vi "LSM9DS1_Read.vi"(0 "LSM9DS1DevRef":T1={"DevStatus"={"status"=FALSE, "code"=0, "source"=""}, "Gyro Offset"={"Xzero"=0.0, "Yzero"=0.0, "Zzero"=0.0}, "StdDev Rates"={"Xsdo"=0.0, "Ysdo"=0.0, "Zsdo"=0.0}, "Reset"=FALSE, "Accel Offset"={"Xzero"=0.0, "Yzero"=0.0, "Zzero"=0.0}, "Motion Thresh"=0.0, "Mag Offset"={"Xzero"=0.0, "Yzero"=0.0, "Zzero"=0.0}, "I2C Bus"=enum."I2C On-Board", "Handle"=0, "Anomaly Thresh"=0.0, "Local Mag"=0.0, "Accel/Gyro_Address"=enum."0x6B", "Accel_Range"=enum."±4g", "Gyro_Range"=enum."±500dps", "Mag_Range"=enum."±2 gauss", "Mag_Address"=enum."0x1E", "accel_active"=FALSE, "gyro_active"=FALSE, "mag_active"=FALSE}, 9 "Reset":bool, 11 "error in (no error)":errorcluster) -> (3 "Filt_Pitch":dbl, 4 "LSM9DS1DevRef Out":T1={"DevStatus"={"status"=FALSE, "code"=0, "source"=""}, "Gyro Offset"={"Xzero"=0.0, "Yzero"=0.0, "Zzero"=0.0}, "StdDev Rates"={"Xsdo"=0.0, "Ysdo"=0.0, "Zsdo"=0.0}, "Reset"=FALSE, "Accel Offset"={"Xzero"=0.0, "Yzero"=0.0, "Zzero"=0.0}, "Motion Thresh"=0.0, "Mag Offset"={"Xzero"=0.0, "Yzero"=0.0, "Zzero"=0.0}, "I2C Bus"=enum."I2C On-Board", "Handle"=0, "Anomaly Thresh"=0.0, "Local Mag"=0.0, "Accel/Gyro_Address"=enum."0x6B", "Accel_Range"=enum."±4g", "Gyro_Range"=enum."±500dps", "Mag_Range"=enum."±2 gauss", "Mag_Address"=enum."0x1E", "accel_active"=FALSE, "gyro_active"=FALSE, "mag_active"=FALSE}, 6 "Gyro":T6, 8 "Accel":T5, 10 "Mag":T4, 15 "error out":errorcluster)   [LabVIEW 2015]
uses:
  <vilib>/Rock Robotics/WPI/I2C/WPI_I2CDevRef.ctl
  <vilib>/Rock Robotics/SystemInterfaces/i2clib/i2c_bus.ctl
  Gyro_TypeDef.ctl
  Accel_TypeDef.ctl
  Mag_TypeDef.ctl
  LSM9DS1DevRef.ctl
panel:
  out "Pitch 2":cluster{"Pitch":dbl, dbl}(graph)
  in  "FIlt_Fact":dbl=1.0
  in  "Filt_Fact":dbl
  in  "In":dbl=0.1
  out "Roll":dbl(knob) scale=-180.0..180.0
  out "Pitch":dbl(knob) scale=-90.0..90.0
  in  "I2CDevRef":T3={"DevStatus"={"status"=FALSE, "code"=0, "source"=""}, "Device Address"=0, "Handle"=0, "I2C Bus"=enum."Invalid"} {"Device Address" format="%.0x"}
  in  "I2CDevRef":T3={"DevStatus"={"status"=FALSE, "code"=0, "source"=""}, "Device Address"=0, "Handle"=0, "I2C Bus"=enum."Invalid"} {"Device Address" format="%.0x"}
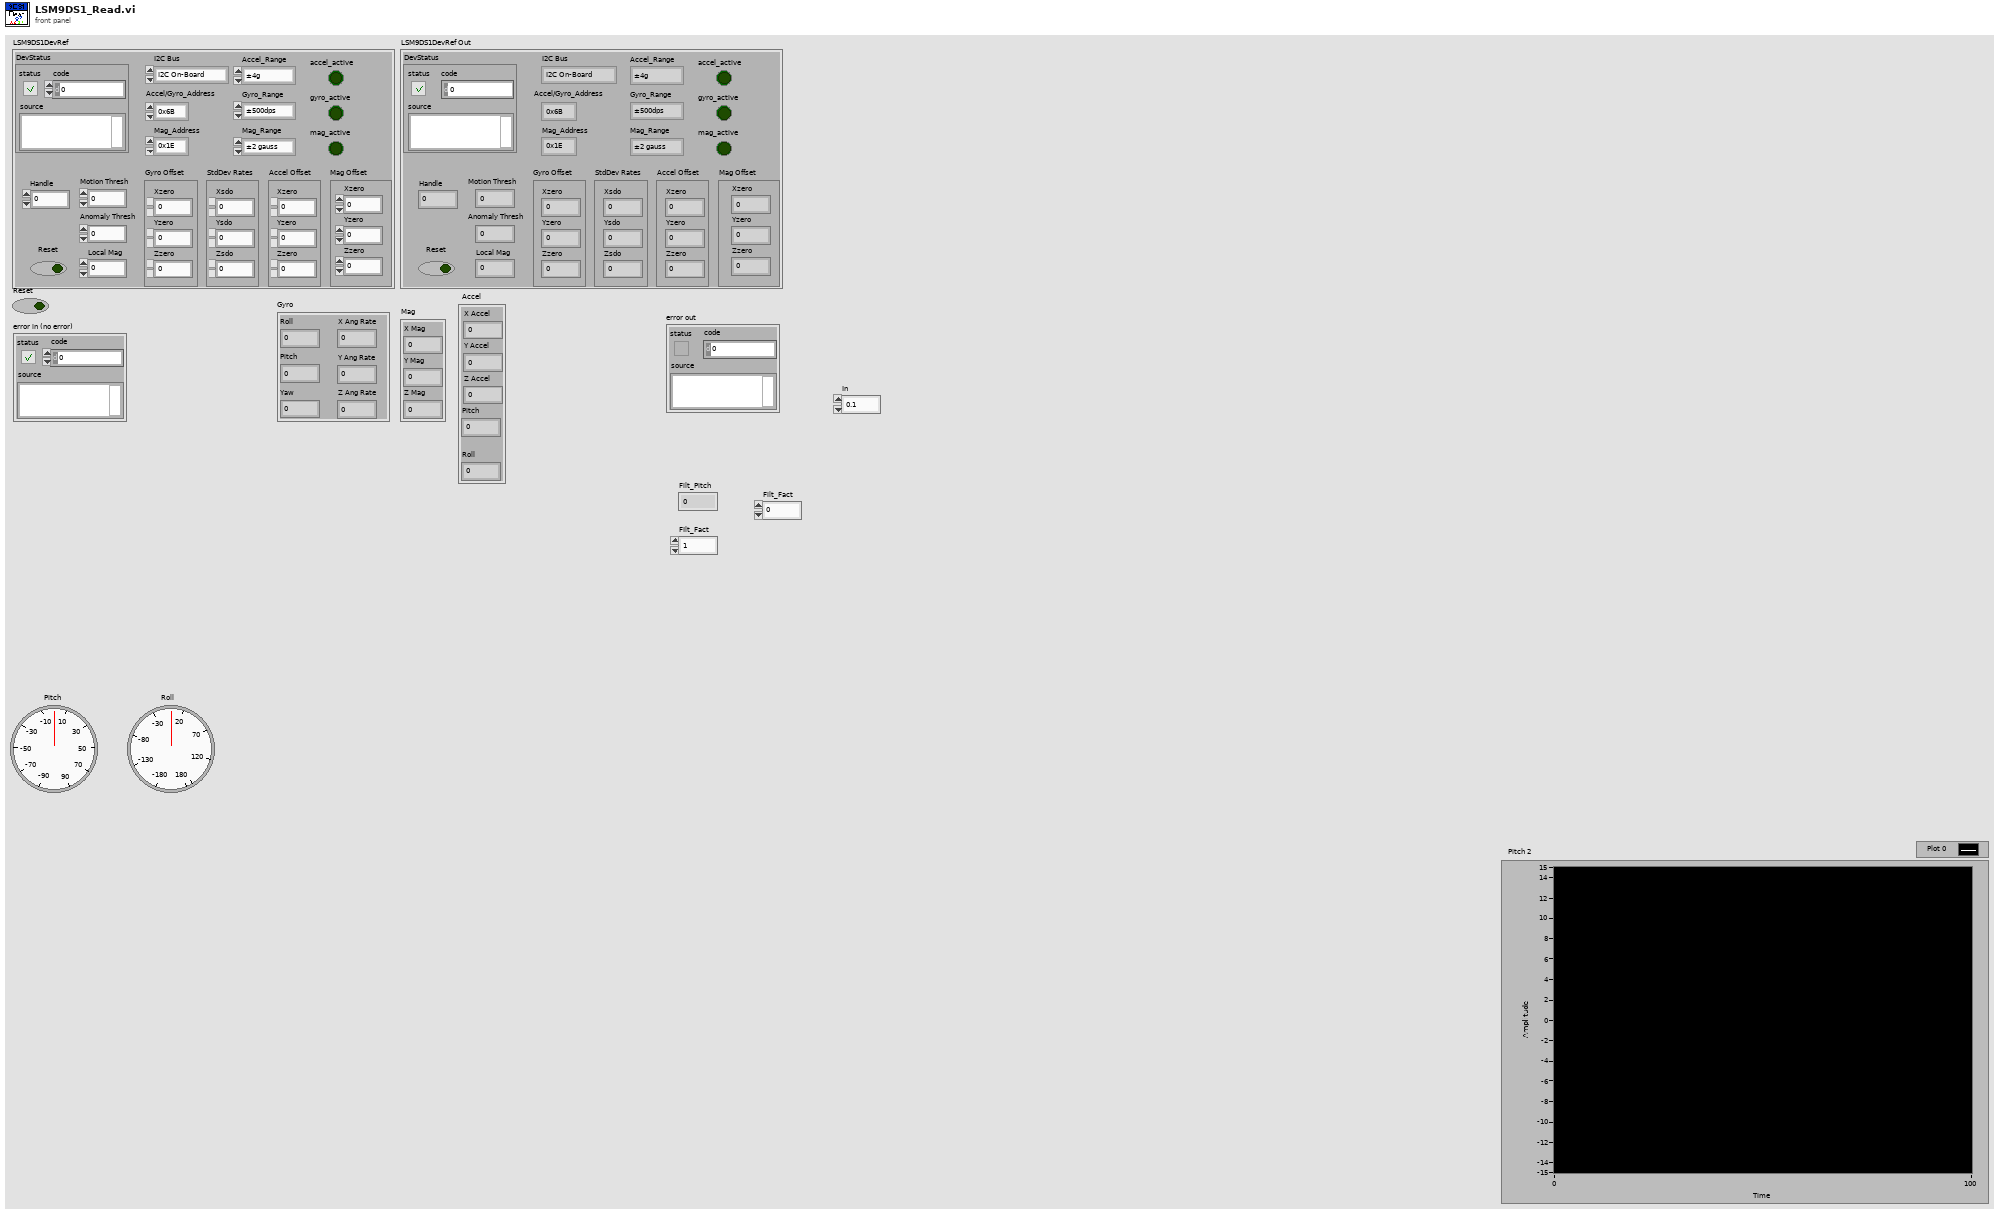
[diagram p1: front panel]
types:
  T1 = typedef "LSM9DS1DevRef.ctl" = cluster{"DevStatus":errorcluster, "Gyro Offset":cluster{"Xzero":dbl, "Yzero":dbl, "Zzero":dbl}, "StdDev Rates":cluster{"Xsdo":dbl, "Ysdo":dbl, "Zsdo":dbl}, "Reset":bool, "Accel Offset":cluster{"Xzero":dbl, "Yzero":dbl, "Zzero":dbl}, "Motion Thresh":dbl, "Mag Offset":cluster{"Xzero":dbl, "Yzero":dbl, "Zzero":dbl}, "I2C Bus":T2, "Handle":i32, "Anomaly Thresh":dbl, "Local Mag":dbl, "Accel/Gyro_Address":enum8{"0x6A", "0x6B"}, "Accel_Range":enum16{"±2g", "±16g", "±4g", "±8g", "disabled"}, "Gyro_Range":enum16{"±245dps", "±500dps", "disabled", "±2000dps"}, "Mag_Range":enum16{"±2 gauss", "±4 gauss", "±8 gauss", "±16 gauss", "disabled"}, "Mag_Address":enum8{"0x1C", "0x1E"}, "accel_active":bool, "gyro_active":bool, "mag_active":bool}
  T2 = typedef "i2c_bus.ctl" = enum16{"I2C On-Board", "I2C MXP", "Invalid"}
  T3 = typedef "WPI_I2CDevRef.ctl" = cluster{"DevStatus":errorcluster, "Device Address":u8, "Handle":i32, "I2C Bus":T2}
  T4 = typedef "Mag_TypeDef.ctl" = cluster{"X Mag":dbl, "Y Mag":dbl, "Z Mag":dbl}
  T5 = typedef "Accel_TypeDef.ctl" = cluster{"X Accel":dbl, "Y Accel":dbl, "Z Accel":dbl, "Pitch":dbl, "Roll":dbl}
  T6 = typedef "Gyro_TypeDef.ctl" = cluster{"Pitch":dbl, "Yaw":dbl, "X Ang Rate":dbl, "Y Ang Rate":dbl, "Z Ang Rate":dbl, "Roll":dbl}
  T7 = enum16{"±2 gauss", "±4 gauss", "±8 gauss", "±16 gauss", "disabled"}
  T8 = enum16{"±245dps", "±500dps", "disabled", "±2000dps"}
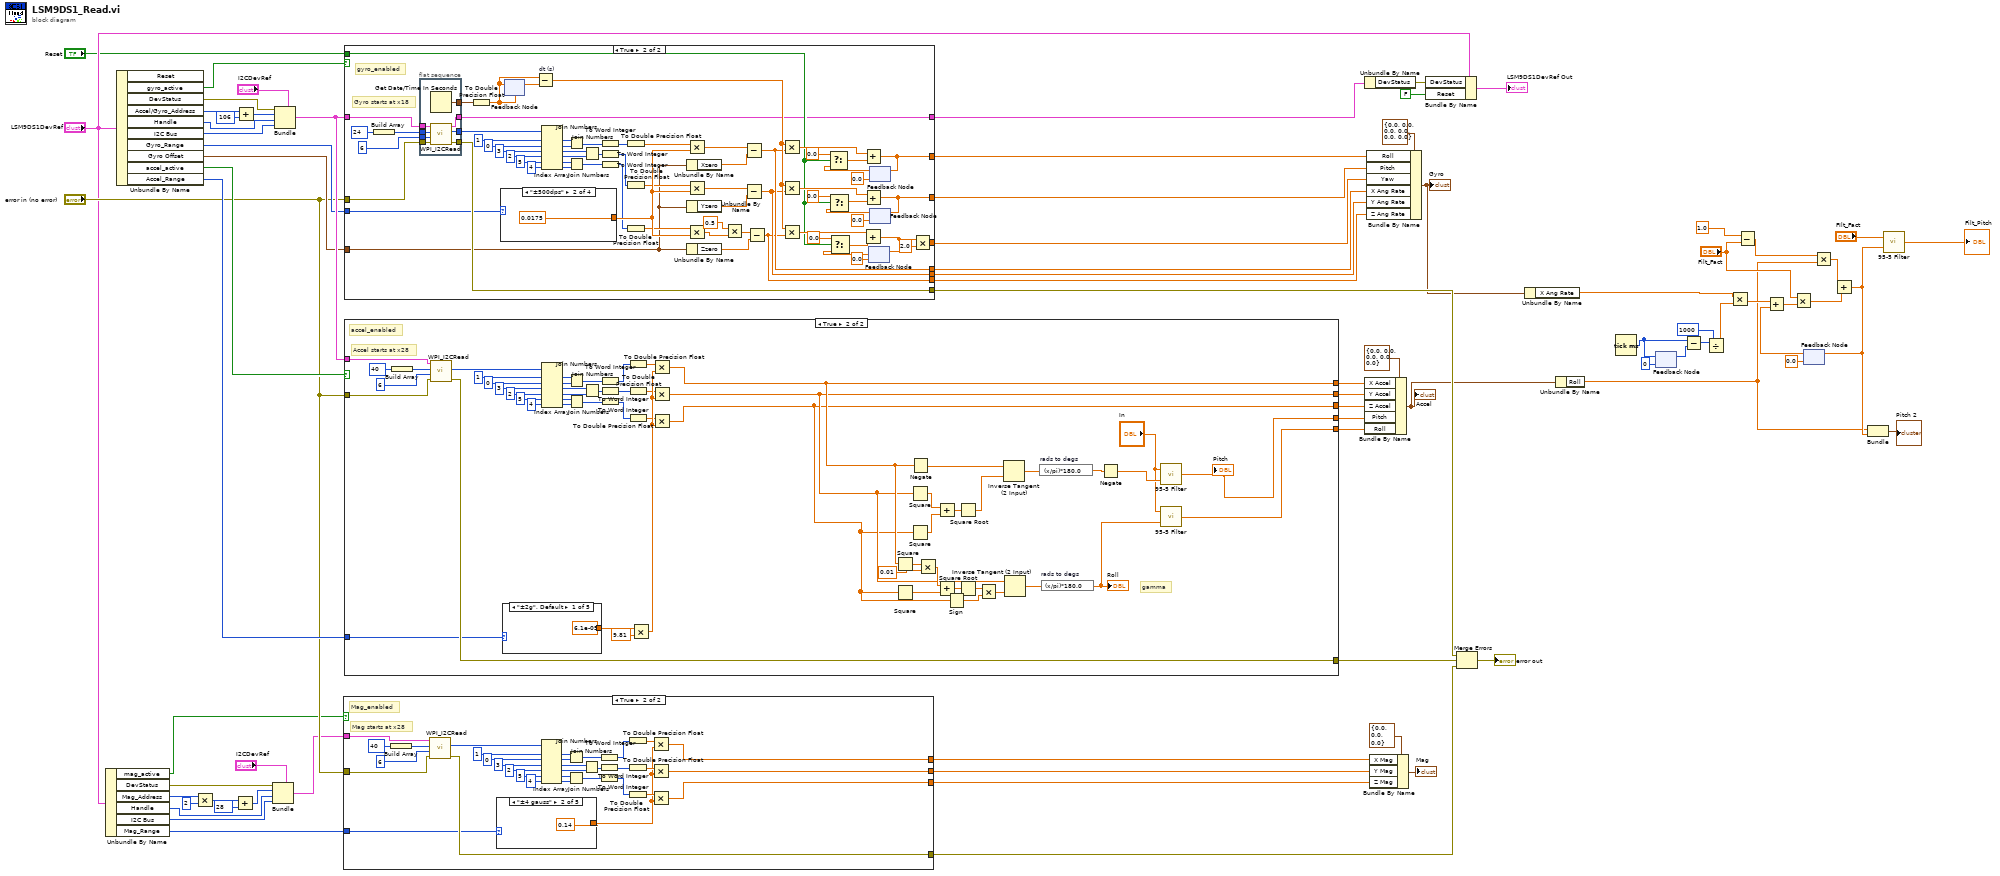
[diagram p0: block diagram]
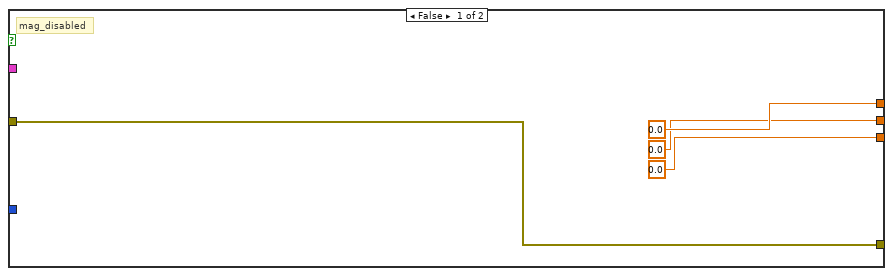
[diagram p2: hidden frame]
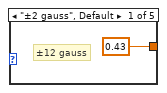
[diagram p3: hidden frame]
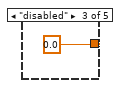
[diagram p4: hidden frame]
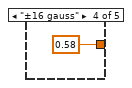
[diagram p5: hidden frame]
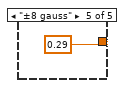
[diagram p6: hidden frame]
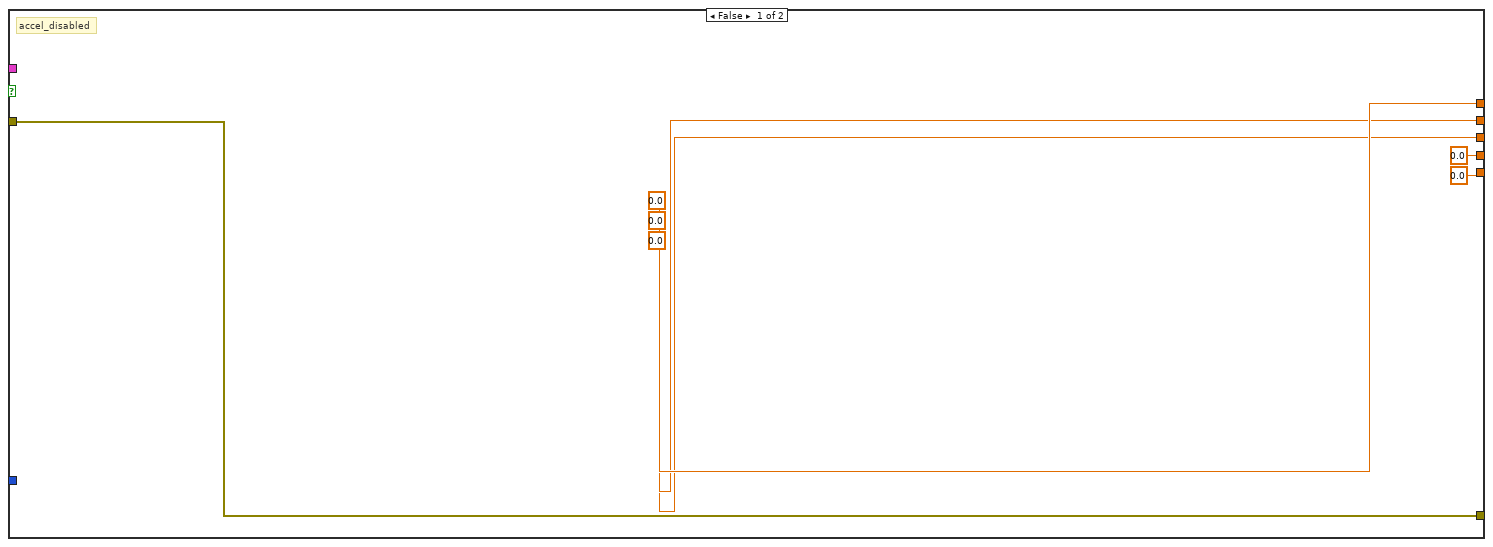
[diagram p7: hidden frame]
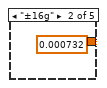
[diagram p8: hidden frame]
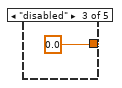
[diagram p9: hidden frame]
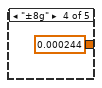
[diagram p10: hidden frame]
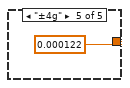
[diagram p11: hidden frame]
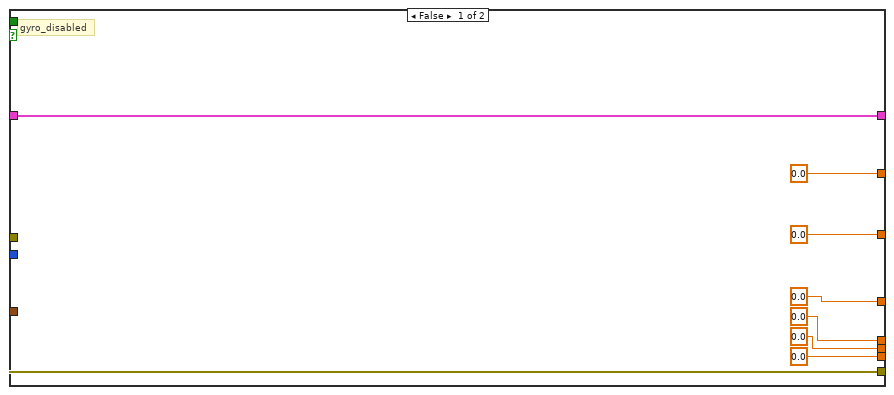
[diagram p12: hidden frame]
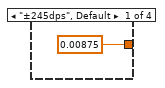
[diagram p13: hidden frame]
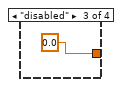
[diagram p14: hidden frame]
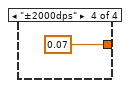
[diagram p15: hidden frame]
diagram:
  n1 = Unbundle By Name("LSM9DS1DevRef") -> ("mag_active"=w42:bool, "DevStatus"=w37:errorcluster, "Mag_Address"=w36:enum8{"0x1C", "0x1E"}, "Handle"=w35:i32, "I2C Bus"=w33:T2, "Mag_Range"=w44:T7)
  n2 = Unbundle By Name("LSM9DS1DevRef") -> ("gyro_active"=w49:bool, "DevStatus"=w56:errorcluster, "Accel/Gyro_Address"=w57:enum8{"0x6A", "0x6B"}, "Handle"=w54:i32, "I2C Bus"=w53:T2, "Gyro_Range"=w50:T8, "Gyro Offset"=w48:cluster{"Xzero":dbl, "Yzero":dbl, "Zzero":dbl}, "accel_active"=w47:bool, "Accel_Range"=w46:enum16{"±2g", "±16g", "±4g", "±8g", "disabled"})  [unwired: 1 out]
  n3 = Multiply(x=w36, y=u8 2) -> (x*y=w40:u8)
  n4 = Add ("Gyro/Accel Slave Address")(x=w40, y=u8 28) -> (x+y=w34:u8)
  n5 = Add ("Gyro/Accel Slave Address")(x=w57, y=u8 106) -> (x+y=w55:u8)
  n6 = Bundle(cluster="I2CDevRef", "DevStatus"=w37, "Device Address"=w34, "Handle"=w35, "I2C Bus"=w33) -> (w41:T3)
  n7 = Bundle(cluster="I2CDevRef", "DevStatus"=w56, "Device Address"=w55, "Handle"=w54, "I2C Bus"=w53) -> (w51:T3)
  n8 = case shown="True" w42 {
    tunnel: [0.0 ("t") w88] -> w63
    tunnel: [0.0 ("t") w87] -> w61
    tunnel: [0.0 ("t") w86] -> w60
    tunnel: [w78 w95] -> w74
    tunnel: w44 -> [_ w85]
    tunnel: w41 -> [_ w83]
    tunnel: "error in (no error)" -> [w78 w82]
    frame False {
      # "mag_disabled"
    }
    frame True {
      # "Mag_enabled"
      # "Mag starts at x28"
      n9 = Build Array(u8 40 ("I2CRegister")) -> (w113:u8[])
      n10 = call <vilib>:"WPI_I2CRead.vi"("error in (no error)"=w82, "I2CBytesToRead"=u8 6, "I2CRegister"=w113, "I2CDevRef"=w83) -> ("error out"=w95:errorcluster, "Data Out"=w96:u8[])  [unwired: 5 in, 1 out]
      n11 = case shown="\"±4 gauss\"" w85 {
        tunnel: [0.43 ("y") 0.14 ("y") 0.0 0.58 ("y") 0.29 ("y")] -> w84
        frame "±2 gauss", Default {
          # "±12 gauss"
        }
        frame "±4 gauss" {
        }
        frame "disabled" {
        }
        frame "±16 gauss" {
        }
        frame "±8 gauss" {
        }
      }
      n12 = Index Array(array=w96, index #1=1 ("index"), index #2=0 ("index"), index #3=3 ("index"), index #4=2 ("index"), index #5=5 ("index"), index #6=4 ("index")) -> (element #1=w106:u8, element #2=w107:u8, element #3=w108:u8, element #4=w109:u8, element #5=w110:u8, element #6=w111:u8)
      n13 = Join Numbers(hi=w106, lo=w107) -> ((hi.lo)=w98:u16)
      n14 = Join Numbers(hi=w110, lo=w111) -> ((hi.lo)=w99:u16)
      n15 = Join Numbers(hi=w108, lo=w109) -> ((hi.lo)=w97:u16)
      n16 = To Word Integer(number=w98) -> (16bit integer=w91:i16)
      n17 = To Word Integer(number=w97) -> (16bit integer=w90:i16)
      n18 = To Word Integer(number=w99) -> (16bit integer=w89:i16)
      n19 = To Double Precision Float(number=w91) -> (double precision float=w92:dbl)
      n20 = To Double Precision Float(number=w90) -> (double precision float=w93:dbl)
      n21 = To Double Precision Float(number=w89) -> (double precision float=w94:dbl)
      n22 = Multiply(x=w92, y=w84) -> (x*y=w88:dbl)
      n23 = Multiply(x=w93, y=w84) -> (x*y=w87:dbl)
      n24 = Multiply(x=w94, y=w84) -> (x*y=w86:dbl)
    }
  }
  n25 = case shown="True" w49 {
    tunnel: w51 -> [w120 w193]
    tunnel: "error in (no error)" -> [w121 w191]
    tunnel: "Reset" -> [_ w147]
    tunnel: [0.0 ("t") w146] -> w73
    tunnel: [0.0 ("t") w145] -> w25
    tunnel: [0.0 ("t") w144] -> w71
    tunnel: [0.0 ("t") w143] -> w70
    tunnel: [0.0 ("t") w142] -> w69
    tunnel: [0.0 ("t") w131] -> w68
    tunnel: [w121 w141] -> w76
    tunnel: w50 -> [_ w140]
    tunnel: w48 -> [_ w133]
    tunnel: [w120 w132] -> w28
    frame False {
      # "gyro_disabled"
    }
    frame True {
      # "gyro_enabled"
      # "Gyro starts at x18"
      n26 = Build Array(u8 24 ("I2CRegister")) -> (w194:u8[])
      n27 = flat-sequence {
        tunnel: w194 -> [w203]
        tunnel: w193 -> [w202]
        tunnel: u8 6 ("I2CBytesToRead") -> [w201]
        tunnel: w191 -> [w200]
        tunnel: [w199] -> w175
        tunnel: [w198] -> w151
        tunnel: [w197] -> w141
        tunnel: [w196] -> w132
        frame #0 {
          n28 = Get Date/Time In Seconds() -> (seconds since 1Jan1904=w198:timestamp)
          n29 = call <vilib>:"WPI_I2CRead.vi"("error in (no error)"=w200, "I2CBytesToRead"=w201, "I2CRegister"=w203, "I2CDevRef"=w202) -> ("error out"=w197:errorcluster, "Data Out"=w199:u8[], "I2CDevRef"=w196:T3)  [unwired: 5 in]
        }
      }
      n30 = To Double Precision Float(number=w151) -> (double precision float=w150:dbl)
      n31 = case shown="\"±500dps\"" w140 {
        tunnel: [0.00875 ("y") 0.0175 ("y") 0.0 ("y") 0.07 ("y")] -> w169
        frame "±245dps", Default {
        }
        frame "±500dps" {
        }
        frame "disabled" {
        }
        frame "±2000dps" {
        }
      }
      n32 = feedback #1(w150) -> (w149:dbl)
      n33 = feedback-in #1(w150) -> ()
      n34 = Subtract "dt (s)"(x=w150, y=w149) -> (x-y=w148:dbl)
      n35 = Index Array(array=w175, index #1=1 ("index"), index #2=0 ("index"), index #3=3 ("index"), index #4=2 ("index"), index #5=5 ("index"), index #6=4 ("index")) -> (element #1=w185:u8, element #2=w186:u8, element #3=w187:u8, element #4=w188:u8, element #5=w189:u8, element #6=w190:u8)
      n36 = Join Numbers(hi=w185, lo=w186) -> ((hi.lo)=w177:u16)
      n37 = Join Numbers(hi=w189, lo=w190) -> ((hi.lo)=w178:u16)
      n38 = Join Numbers(hi=w187, lo=w188) -> ((hi.lo)=w176:u16)
      n39 = To Word Integer(number=w177) -> (16bit integer=w138:i16)
      n40 = To Word Integer(number=w176) -> (16bit integer=w137:i16)
      n41 = To Word Integer(number=w178) -> (16bit integer=w135:i16)
      n42 = To Double Precision Float(number=w138) -> (double precision float=w139:dbl)
      n43 = To Double Precision Float(number=w137) -> (double precision float=w136:dbl)
      n44 = To Double Precision Float(number=w135) -> (double precision float=w134:dbl)
      n45 = Multiply(x=w139, y=w169) -> (x*y=w171:dbl)
      n46 = Unbundle By Name(w133) -> ("Xzero"=w170:dbl)
      n47 = Multiply(x=w136, y=w169) -> (x*y=w173:dbl)
      n48 = Unbundle By Name(w133) -> ("Yzero"=w172:dbl)
      n49 = Multiply(x=w134, y=w169) -> (x*y=w129:dbl)
      n50 = Unbundle By Name(w133) -> ("Zzero"=w174:dbl)
      n51 = Multiply(x=0.5 ("y"), y=w129) -> (x*y=w130:dbl)
      n52 = Subtract(x=w171, y=w170) -> (x-y=w143:dbl)
      n53 = Subtract(x=w173, y=w172) -> (x-y=w142:dbl)
      n54 = Subtract(x=w130, y=w174) -> (x-y=w131:dbl)
      n55 = Multiply(x=w148, y=w143) -> (x*y=w164:dbl)
      n56 = Multiply(x=w148, y=w142) -> (x*y=w160:dbl)
      n57 = Multiply(x=w148, y=w131) -> (x*y=w154:dbl)
      n58 = feedback #2(0.0) -> (w157:dbl)
      n59 = Select(t=0.0, s=w147, f=w157) -> (s? t:f=w156:dbl)
      n60 = Add(x=w154, y=w156) -> (x+y=w153:dbl)
      n61 = feedback-in #2(w153) -> ()
      n62 = feedback #3(0.0) -> (w165:dbl)
      n63 = Select(t=0.0, s=w147, f=w165) -> (s? t:f=w166:dbl)
      n64 = Add(x=w164, y=w166) -> (x+y=w146:dbl)
      n65 = feedback-in #3(w146) -> ()
      n66 = feedback #4(0.0) -> (w159:dbl)
      n67 = Select(t=0.0, s=w147, f=w159) -> (s? t:f=w161:dbl)
      n68 = Add(x=w160, y=w161) -> (x+y=w145:dbl)
      n69 = feedback-in #4(w145) -> ()
      n70 = Multiply(x=w153, y=2.0) -> (x*y=w144:dbl)
    }
  }
  n71 = case shown="True" w47 {
    tunnel: [0.0 ("t") w222] -> w66
    tunnel: [0.0 ("t") w221] -> w65
    tunnel: [0.0 ("t") w220] -> w64
    tunnel: [w212 w250] -> w75
    tunnel: "error in (no error)" -> [w212 w249]
    tunnel: w46 -> [_ w239]
    tunnel: w51 -> [_ w238]
    tunnel: [0.0 w218] -> w24
    tunnel: [0.0 w214] -> w26
    frame False {
      # "accel_disabled"
    }
    frame True {
      # "gamma"
      # "accel_enabled"
      # "Accel starts at x28"
      n72 = Build Array(u8 40 ("I2CRegister")) -> (w268:u8[])
      n73 = call <vilib>:"WPI_I2CRead.vi"("error in (no error)"=w249, "I2CBytesToRead"=u8 6, "I2CRegister"=w268, "I2CDevRef"=w238) -> ("error out"=w250:errorcluster, "Data Out"=w251:u8[])  [unwired: 5 in, 1 out]
      n74 = case shown="\"±2g\", Default" w239 {
        tunnel: [6.1e-05 ("y") 0.000732 ("y") 0.0 0.000244 ("y") 0.000122 ("y")] -> w248
        frame "±2g", Default {
        }
        frame "±16g" {
        }
        frame "disabled" {
        }
        frame "±8g" {
        }
        frame "±4g" {
        }
      }
      n75 = Index Array(array=w251, index #1=1 ("index"), index #2=0 ("index"), index #3=3 ("index"), index #4=2 ("index"), index #5=5 ("index"), index #6=4 ("index")) -> (element #1=w261:u8, element #2=w262:u8, element #3=w263:u8, element #4=w264:u8, element #5=w265:u8, element #6=w266:u8)
      n76 = Join Numbers(hi=w261, lo=w262) -> ((hi.lo)=w253:u16)
      n77 = Join Numbers(hi=w265, lo=w266) -> ((hi.lo)=w254:u16)
      n78 = Join Numbers(hi=w263, lo=w264) -> ((hi.lo)=w252:u16)
      n79 = To Word Integer(number=w253) -> (16bit integer=w242:i16)
      n80 = To Word Integer(number=w252) -> (16bit integer=w241:i16)
      n81 = To Word Integer(number=w254) -> (16bit integer=w240:i16)
      n82 = To Double Precision Float(number=w242) -> (double precision float=w243:dbl)
      n83 = To Double Precision Float(number=w241) -> (double precision float=w244:dbl)
      n84 = To Double Precision Float(number=w240) -> (double precision float=w245:dbl)
      n85 = Multiply(x=w248, y=9.81) -> (x*y=w246:dbl)
      n86 = Multiply(x=w243, y=w246) -> (x*y=w222:dbl)
      n87 = Multiply(x=w244, y=w246) -> (x*y=w221:dbl)
      n88 = Multiply(x=w245, y=w246) -> (x*y=w220:dbl)
      n89 = Square(x=w222) -> (x^2=w232:dbl)
      n90 = Square(x=w220) -> (x^2=w229:dbl)
      n91 = Square(x=w221) -> (x^2=w225:dbl)
      n92 = Square(x=w220) -> (x^2=w226:dbl)
      n93 = Negate(x=w222) -> (-x=w234:dbl)
      n94 = Multiply(x=w232, y=0.01 ("u 2")) -> (x*y=w233:dbl)
      n95 = Add(x=w225, y=w226) -> (x+y=w227:dbl)
      n96 = Add(x=w233, y=w229) -> (x+y=w228:dbl)
      n97 = Sign(1:w220) -> (0:w231:dbl)
      n98 = Square Root(x=w227) -> (sqrt(x)=w235:dbl)
      n99 = Square Root(x=w228) -> (sqrt(x)=w230:dbl)
      n100 = Multiply(x=w230, y=w231) -> (x*y=w236:dbl)
      n101 = Inverse Tangent (2 Input)(1:w235, 2:w234) -> (0:w223:dbl)
      n102 = Inverse Tangent (2 Input)(1:w236, 2:w221) -> (0:w224:dbl)
      n103 = expression code="(x/pi)*180.0" "rads to degs"(w223) -> (w219:dbl)
      n104 = expression code="(x/pi)*180.0" "rads to degs"(w224) -> (w215:dbl)
      "Roll" <- w215
      n105 = Negate(x=w219) -> (-x=w217:dbl)
      n106 = call "95-5 Filter.vi"("In"=w217, "Percent"="In") -> ("Out"=w218:dbl)
      "Pitch" <- w218
      n107 = call "95-5 Filter.vi"("In"=w215, "Percent"="In") -> ("Out"=w214:dbl)
    }
  }
  n108 = Unbundle By Name(w28) -> ("DevStatus"=w32:errorcluster)
  n109 = Bundle By Name(cluster=T5 {"X Accel"=0.0, "Y Accel"=0.0, "Z Accel"=0.0, "Pitch"=0.0, "Roll"=0.0} ("Accel"), "X Accel"=w66, "Y Accel"=w65, "Z Accel"=w64, "Pitch"=w24, "Roll"=w26) -> (w5:T5)
  "Accel" <- w5
  n110 = Bundle By Name(cluster=T6 {"Pitch"=0.0, "Yaw"=0.0, "X Ang Rate"=0.0, "Y Ang Rate"=0.0, "Z Ang Rate"=0.0, "Roll"=0.0} ("Gyro"), "Roll"=w73, "Pitch"=w25, "Yaw"=w71, "X Ang Rate"=w70, "Y Ang Rate"=w69, "Z Ang Rate"=w68) -> (w4:T6)
  "Gyro" <- w4
  n111 = Bundle By Name(cluster=T4 {"X Mag"=0.0, "Y Mag"=0.0, "Z Mag"=0.0} ("Mag"), "X Mag"=w63, "Y Mag"=w61, "Z Mag"=w60) -> (→"Mag":T4)
  n112 = Bundle By Name(cluster="LSM9DS1DevRef", "DevStatus"=w32, "Reset"=FALSE ("Fast")) -> (→"LSM9DS1DevRef Out":T1)
  n113 = Merge Errors(w76, w75, w74) -> (→"error out":errorcluster)
  n114 = Unbundle By Name(w4) -> ("X Ang Rate"=w3:dbl)
  n115 = Unbundle By Name(w5) -> ("Roll"=w2:dbl)
  n116 = Tick Count (ms)() -> (millisecond timer value=w9:u32)
  n117 = feedback #5(u32 0 ("millisecond timer value")) -> (w13:u32)
  n118 = feedback-in #5(w9) -> ()
  n119 = Subtract(x=w9, y=w13) -> (x-y=w12:u32)
  n120 = Divide(x=w12, y=u32 1000) -> (x/y=w10:dbl)
  n121 = Multiply(x=w3, y=w10) -> (x*y=w22:dbl)
  n122 = Subtract(x=1.0, y="Filt_Fact") -> (x-y=w19:dbl)
  n123 = feedback #6(0.0) -> (w16:dbl)
  n124 = Add(x=w22, y=w16) -> (x+y=w21:dbl)
  n125 = Multiply(x="Filt_Fact", y=w21) -> (x*y=w17:dbl)
  n126 = Multiply(x=w19, y=w2) -> (x*y=w18:dbl)
  n127 = Add(x=w18, y=w17) -> (x+y=w6:dbl)
  n128 = feedback-in #6(w6) -> ()
  n129 = Bundle("Roll"=w2, w6) -> (→"Pitch 2":cluster{"Roll":dbl, dbl})  [unwired: 1 in]
  n130 = call "95-5 Filter.vi"("In"=w6, "Percent"="FIlt_Fact") -> ("Out"=→"Filt_Pitch":dbl)
